vi "niRFUtil WFM Unwrap Phase (real array).vi"(0 "Phase In (rad)":T1 min=0 max=127 format="%.2f") -> (4 "Phase Out (rad)":T1 min=0 max=127 format="%.2f")   [LabVIEW 2015, in "niRFUtil.lvlib"]
uses:
  niRFUtil.lvlib
  Includes/niRFUtil INC Real Array.ctl
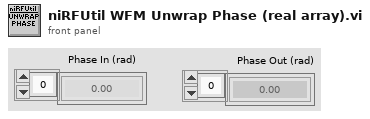
[diagram p1: front panel]
types:
  T1 = typedef "niRFUtil.lvlib/niRFUtil INC Real Array.ctl" = sgl[]
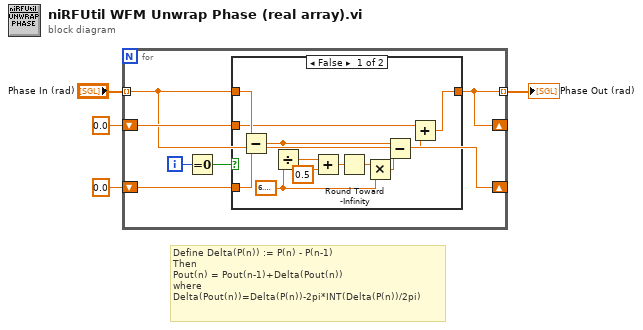
[diagram p0: block diagram]
diagram:
  # "Define Delta(P(n)) := P(n) - P(n-1)\nThen\nPout(n) = Pout(n-1)+Delta(Pout(n))\nwhere\nDelta(Pout(n))=Delta(P(n))-2pi*INT(Delta(P(n))/2pi)"
  n1 = for {
    tunnel: "Phase In (rad)" -> [w5] mode=indexing
    tunnel: [w7] -> w2 mode=indexing
    shift-right: [w7] -> _
    shift-left: sgl 0.0 -> [w8]
    shift-right: [w5] -> _
    shift-left: sgl 0.0 -> [w6]
    i -> [w9]
    n2 = Equal To 0?(x=w9) -> (x = 0?=w10:bool)
    n3 = case shown="False" w10 {
      tunnel: w8 -> [w16 _]
      tunnel: w5 -> [w22 w23]
      tunnel: [w15 w23] -> w7
      tunnel: w6 -> [w21 _]
      frame False {
        w20 = sgl 6.2831855
        n4 = Subtract(x=w22, y=w21) -> (x-y=w18:sgl)
        n5 = Divide(x=w18, y=w20) -> (x/y=w14:sgl)
        n6 = Add(x=w14, y=sgl 0.5) -> (x+y=w12:sgl)
        n7 = Round Toward -Infinity(1:w12) -> (0:w11:sgl)
        n8 = Multiply(x=w11, y=w20) -> (x*y=w19:sgl)
        n9 = Subtract(x=w18, y=w19) -> (x-y=w17:sgl)
        n10 = Add(x=w16, y=w17) -> (x+y=w15:sgl)
      }
      frame True {
      }
    }
  }
  "Phase Out (rad)" <- w2
